vi "Gen_Random_Dumping_Sine.vi"() -> (3 "data":dbl[](graph))   [LabVIEW 2020]
uses:
  <vilib>/Analysis/1siggen.llb/Ramp Pattern by Samples.vi
  <vilib>/measure/NI_MABase.lvlib
  <vilib>/Analysis/NI_AALBase.lvlib
panel:
  out "data 2":dbl[](graph)
  in  "Duration":dbl=50.0 format="%#_13g"
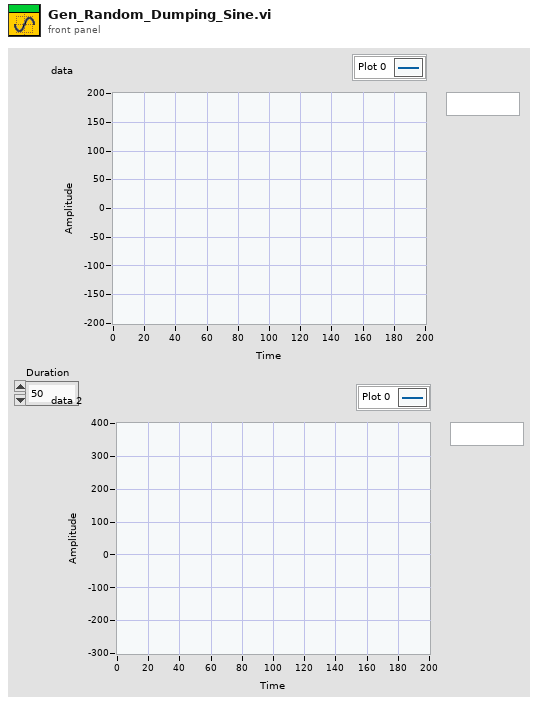
[diagram p1: front panel]
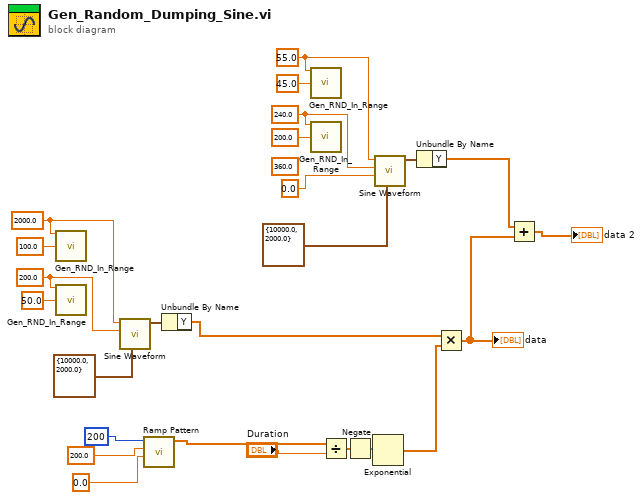
[diagram p0: block diagram]
diagram:
  w3 = 55.0 ("frequency")
  w2 = 240.0 ("amplitude")
  (unwired) 360.0 ("phase(digree)")
  w4 = 2000.0 ("frequency")
  w5 = 200.0 ("amplitude")
  n1 = call "Gen_RND_In_Range.vi"("Upper Bound"=w4, "Lower Bound"=100.0 ("Variation%")) -> ()  [unwired: 13 in, 1 out]
  n2 = call "Gen_RND_In_Range.vi"("Upper Bound"=w5, "Lower Bound"=50.0 ("variation")) -> ()  [unwired: 13 in, 1 out]
  n3 = call <vilib>:"Sine Waveform.vi"("sampling info"=cluster{"Fs":dbl, "#s":dbl} {"Fs"=10000.0, "#s"=2000.0} ("sampling info for sine"), "amplitude"=w5, "frequency"=w4) -> ("signal out"=w25:waveform(dbl))  [unwired: 7 in, 1 out]
  n4 = call-poly <vilib>:"Ramp Pattern.vi"("start"=0.0 ("end"), "end"=200.0, "samples"=200) -> ("Ramp Pattern"=w20:dbl[])  [unwired: 7 in, 1 out]
  n5 = Unbundle By Name(w25) -> ("Y"=w14:dbl[])
  n6 = call "Gen_RND_In_Range.vi"("Upper Bound"=w3, "Lower Bound"=45.0 ("Variation%")) -> ()  [unwired: 13 in, 1 out]
  n7 = call "Gen_RND_In_Range.vi"("Upper Bound"=w2, "Lower Bound"=200.0 ("variation")) -> ()  [unwired: 13 in, 1 out]
  n8 = Divide(x=w20, y="Duration") -> (x/y=w17:dbl[])
  n9 = Negate(x=w17) -> (-x=w13:dbl[])
  n10 = Exponential(1:w13) -> (0:w15:dbl[])
  n11 = call <vilib>:"Sine Waveform.vi"("sampling info"=cluster{"Fs":dbl, "#s":dbl} {"Fs"=10000.0, "#s"=2000.0} ("sampling info for sine"), "phase"=0.0 ("Range"), "amplitude"=w2, "frequency"=w3) -> ("signal out"=w12:waveform(dbl))  [unwired: 6 in, 1 out]
  n12 = Unbundle By Name(w12) -> ("Y"=w8:dbl[])
  n13 = Multiply(x=w14, y=w15) -> (x*y=w7:dbl[])
  "data" <- w7
  n14 = Add(x=w8, y=w7) -> (x+y=→"data 2":dbl[])
